vi "Set data waveform.vi"(8 "data":dbl, 9 "Waveform data":waveform(dbl), 11 "waveform datapoints":dbl) -> (0 "SubWaveform":waveform(dbl), 1 "Appened Waveform":waveform(dbl))   [LabVIEW 2020]
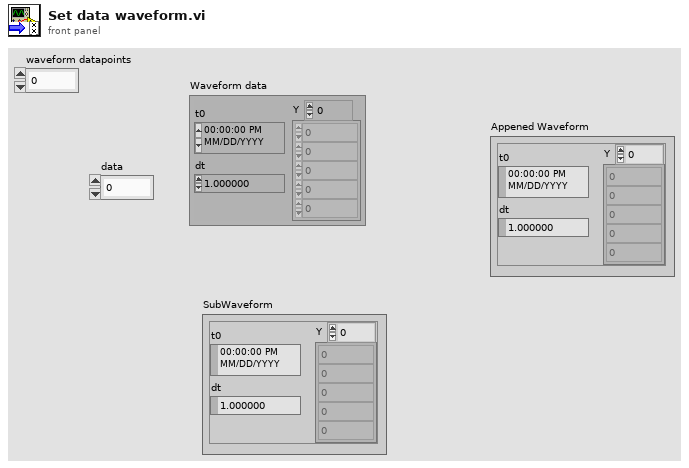
[diagram p1: front panel]
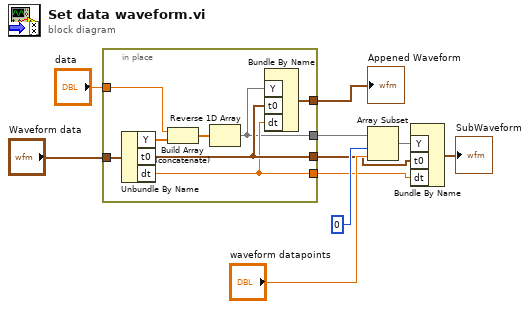
[diagram p0: block diagram]
diagram:
  n1 = in-place {
    in-place-border: "Waveform data" -> [w18]
    in-place-border: "data" -> [w16]
    in-place-border: [w15] -> w8
    in-place-border: [w11] -> w5
    in-place-border: [w14] -> w3
    in-place-border: [w13] -> w2
    n2 = Unbundle By Name(w18) -> ("Y"=w17:dbl[], "t0"=w14:timestamp, "dt"=w13:dbl)
    n3 = Build Array (concatenate)(w16, w17) -> (w12:dbl[])
    n4 = Reverse 1D Array(array=w12) -> (reversed array=w11:dbl[])
    n5 = Bundle By Name("Y"=w11, "t0"=w14, "dt"=w13) -> (w15:waveform(dbl))  [unwired: 1 in]
  }
  "Appened Waveform" <- w8
  n6 = Array Subset(array=w5, index=0, length="waveform datapoints") -> (w4:dbl[])
  n7 = Bundle By Name("Y"=w4, "t0"=w3, "dt"=w2) -> (→"SubWaveform":waveform(dbl))  [unwired: 1 in]
